vi "applyNewPGAGain.vi"(8 "error in (no error)":errorcluster, 10 "Preamplifier Gain":u8 min=1, 11 "Model in":refnum<class "Model.lvclass">) -> (0 "error out":errorcluster, 3 "Model out":refnum<class "Model.lvclass">)   [LabVIEW 2013, in "Model.lvclass"]
uses:
  Model.lvclass
  Model.lvclass/Model.ctl
  <userlib>/Common/ILC/ILC/ILC.lvclass
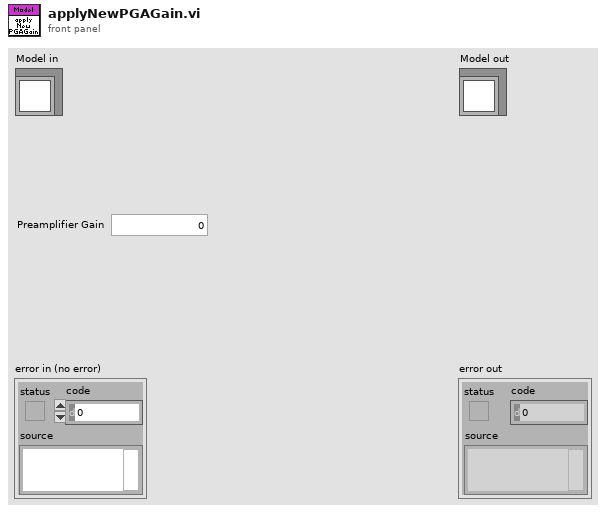
[diagram p1: front panel]
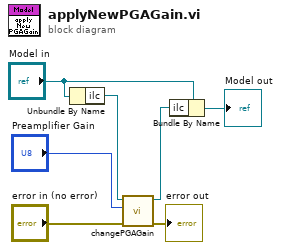
[diagram p0: block diagram]
diagram:
  n1 = Unbundle By Name("Model in") -> ("ilc"=w7:refnum<class "ILC.lvclass">)
  n2 = call <userlib>:"changePGAGain.vi"("error in (no error)"="error in (no error)", "Preamplifier Gain"="Preamplifier Gain", "ILC in"=w7) -> ("error out"=→"error out":errorcluster, "ILC out"=w6:refnum<class "ILC.lvclass">)  [unwired: 7 in]
  n3 = Bundle By Name(cluster="Model in", "ilc"=w6) -> (→"Model out":refnum<class "Model.lvclass">)
